vi "readTelemetryForceActuatorData.vi"(8 "error in (no error)":errorcluster, 10 "Parser":refnum<class "U8ArrayParserAutoIndexing.lvclass">, 11 "M1M3SAL in":refnum<class "M1M3SAL.lvclass">) -> (0 "error out":errorcluster, 2 "EventSummaryState":variant, 3 "M1M3SAL out":refnum<class "M1M3SAL.lvclass">)   [LabVIEW 2016, in "M1M3SupportCommunicator.lvlib" / "M1M3SAL.lvclass"]
uses:
  M1M3SAL.lvclass
  Common_RT_Utilities/U8ArrayParserAutoIndexing/U8ArrayParserAutoIndexing.lvclass
  DataTypes/Topics/TelemetryForceActuatorData.ctl
  DataTypes/Topics/Parts/Timestamp.ctl
  DataTypes/Topics/M1M3SupportTopics.lvlib
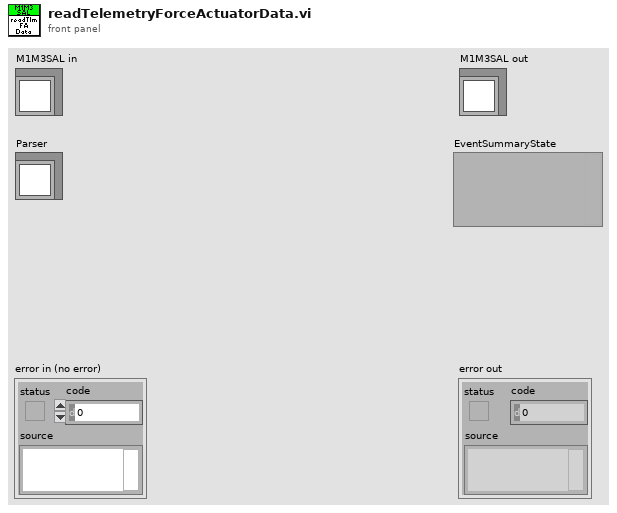
[diagram p1: front panel]
types:
  T1 = typedef "M1M3SupportTopics.lvlib/TelemetryForceActuatorData.ctl" = cluster{"Timestamp":T2, "SlewFlagCommanded":bool[], "XSetpointCommanded":dbl[], "YSetpointCommanded":dbl[], "ZSetpointCommanded":dbl[], "XForce":sgl[], "YForce":sgl[], "ZForce":sgl[], "ILCFault":bool[], "DCAFault":bool[], "BroadcastCounter":u8[]}
  T2 = typedef "M1M3SupportTopics.lvlib/Timestamp.ctl" = dbl
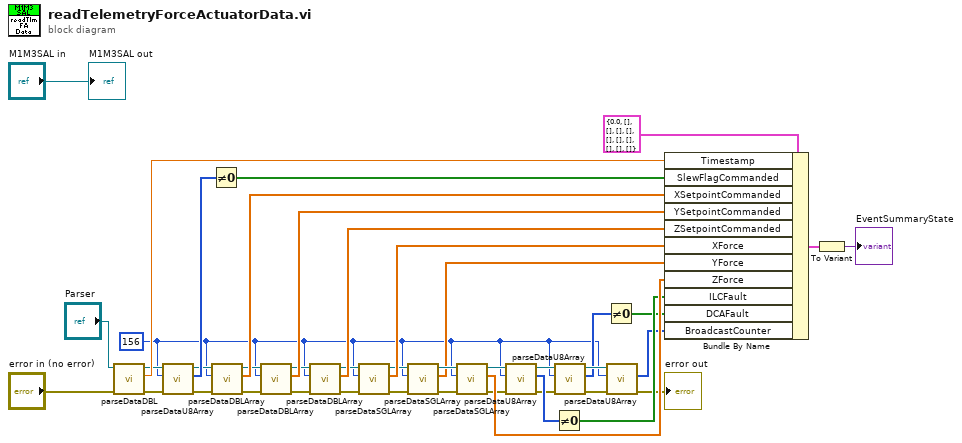
[diagram p0: block diagram]
diagram:
  w1 = 156 ("Length")
  n1 = call "parseDataDBL.vi"("error in (no error)"="error in (no error)", "U8ArrayParserAutoIndexing in"="Parser") -> ("error out"=w36:errorcluster, "Data"=w32:dbl, "U8ArrayParserAutoIndexing out"=w9:refnum<class "U8ArrayParserAutoIndexing.lvclass">)  [unwired: 7 in]
  n2 = call "parseDataU8Array.vi"("U8ArrayParserAutoIndexing in"=w9, "Length"=w1, "error in (no error)"=w36) -> ("U8ArrayParserAutoIndexing out"=w8:refnum<class "U8ArrayParserAutoIndexing.lvclass">, "Data"=w31:u8[], "error out"=w35:errorcluster)  [unwired: 5 in]
  n3 = Not Equal To 0?(x=w31) -> (x != 0?=w30:bool[])
  n4 = call "parseDataDBLArray.vi"("U8ArrayParserAutoIndexing in"=w8, "Length"=w1, "error in (no error)"=w35) -> ("U8ArrayParserAutoIndexing out"=w7:refnum<class "U8ArrayParserAutoIndexing.lvclass">, "Data"=w29:dbl[], "error out"=w34:errorcluster)  [unwired: 5 in]
  n5 = call "parseDataDBLArray.vi"("U8ArrayParserAutoIndexing in"=w7, "Length"=w1, "error in (no error)"=w34) -> ("U8ArrayParserAutoIndexing out"=w6:refnum<class "U8ArrayParserAutoIndexing.lvclass">, "Data"=w28:dbl[], "error out"=w33:errorcluster)  [unwired: 5 in]
  n6 = call "parseDataDBLArray.vi"("U8ArrayParserAutoIndexing in"=w6, "Length"=w1, "error in (no error)"=w33) -> ("U8ArrayParserAutoIndexing out"=w5:refnum<class "U8ArrayParserAutoIndexing.lvclass">, "Data"=w27:dbl[], "error out"=w24:errorcluster)  [unwired: 5 in]
  n7 = call "parseDataSGLArray.vi"("U8ArrayParserAutoIndexing in"=w5, "Length"=w1, "error in (no error)"=w24) -> ("U8ArrayParserAutoIndexing out"=w4:refnum<class "U8ArrayParserAutoIndexing.lvclass">, "Data"=w22:sgl[], "error out"=w23:errorcluster)  [unwired: 5 in]
  n8 = call "parseDataSGLArray.vi"("U8ArrayParserAutoIndexing in"=w4, "Length"=w1, "error in (no error)"=w23) -> ("U8ArrayParserAutoIndexing out"=w26:refnum<class "U8ArrayParserAutoIndexing.lvclass">, "Data"=w21:sgl[], "error out"=w25:errorcluster)  [unwired: 5 in]
  n9 = call "parseDataSGLArray.vi"("U8ArrayParserAutoIndexing in"=w26, "Length"=w1, "error in (no error)"=w25) -> ("U8ArrayParserAutoIndexing out"=w3:refnum<class "U8ArrayParserAutoIndexing.lvclass">, "Data"=w20:sgl[], "error out"=w11:errorcluster)  [unwired: 5 in]
  n10 = call "parseDataU8Array.vi"("U8ArrayParserAutoIndexing in"=w3, "Length"=w1, "error in (no error)"=w11) -> ("U8ArrayParserAutoIndexing out"=w2:refnum<class "U8ArrayParserAutoIndexing.lvclass">, "Data"=w17:u8[], "error out"=w12:errorcluster)  [unwired: 5 in]
  n11 = Not Equal To 0?(x=w17) -> (x != 0?=w16:bool[])
  n12 = call "parseDataU8Array.vi"("U8ArrayParserAutoIndexing in"=w2, "Length"=w1, "error in (no error)"=w12) -> ("U8ArrayParserAutoIndexing out"=w19:refnum<class "U8ArrayParserAutoIndexing.lvclass">, "Data"=w15:u8[], "error out"=w18:errorcluster)  [unwired: 5 in]
  n13 = Not Equal To 0?(x=w15) -> (x != 0?=w14:bool[])
  n14 = call "parseDataU8Array.vi"("U8ArrayParserAutoIndexing in"=w19, "Length"=w1, "error in (no error)"=w18) -> ("Data"=w13:u8[], "error out"=→"error out":errorcluster)  [unwired: 5 in, 1 out]
  n15 = Bundle By Name(cluster=T1 {"Timestamp"=0.0, "SlewFlagCommanded"=[], "XSetpointCommanded"=[], "YSetpointCommanded"=[], "ZSetpointCommanded"=[], "XForce"=[], "YForce"=[], "ZForce"=[], "ILCFault"=[], "DCAFault"=[], "BroadcastCounter"=[]} ("TelemetryForceActuatorData"), "Timestamp"=w32, "SlewFlagCommanded"=w30, "XSetpointCommanded"=w29, "YSetpointCommanded"=w28, "ZSetpointCommanded"=w27, "XForce"=w22, "YForce"=w21, "ZForce"=w20, "ILCFault"=w16, "DCAFault"=w14, "BroadcastCounter"=w13) -> (w41:T1)
  n16 = To Variant(anything=w41) -> (Variant=→"EventSummaryState":variant)
  "M1M3SAL out" <- "M1M3SAL in"
